vi "User32.DestroyWindow.vi"(0 "HWnd":i32, 11 "ErrorIn":errorcluster) -> (15 "ErrorOut":errorcluster)   [LabVIEW 2021]
uses:
  user32.dll
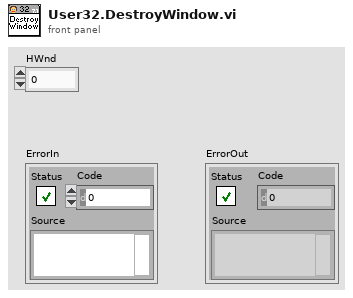
[diagram p1: front panel]
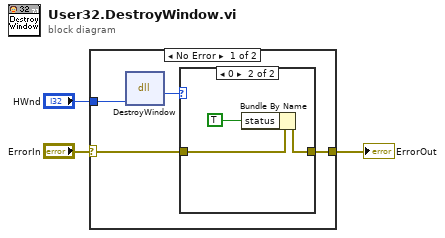
[diagram p0: block diagram]
diagram:
  n1 = case shown="No Error" "ErrorIn" {
    selector: "ErrorIn" -> [w7 w12]
    tunnel: "HWnd" -> [w5 _]
    tunnel: [w6 w12] -> w2
    frame No Error {
      n2 = dll-call lib="user32.dll" fn="DestroyWindow"("hWnd"=w5) -> (w4:u8)  [unwired: 4 in, 2 out]
      n3 = case shown="0" w4 {
        tunnel: w7 -> [w8 w11]
        tunnel: [w8 w10] -> w6
        frame Default {
        }
        frame 0 {
          n4 = Bundle By Name(cluster=w11, "status"=TRUE) -> (w10:errorcluster)
        }
      }
    }
    frame Error {
    }
  }
  "ErrorOut" <- w2
